vi "古田污水厂流程自动启动.vi"(11 "参数":cluster{"是否启用仪器":bool}) -> ()   [LabVIEW 2016, in "PLC.lvlib"]
uses:
  PLC.lvlib
panel:
  out "枚举":enum16{"初始化", "采配水启动", "等待", "配水", "排水", "结束"}(ring)
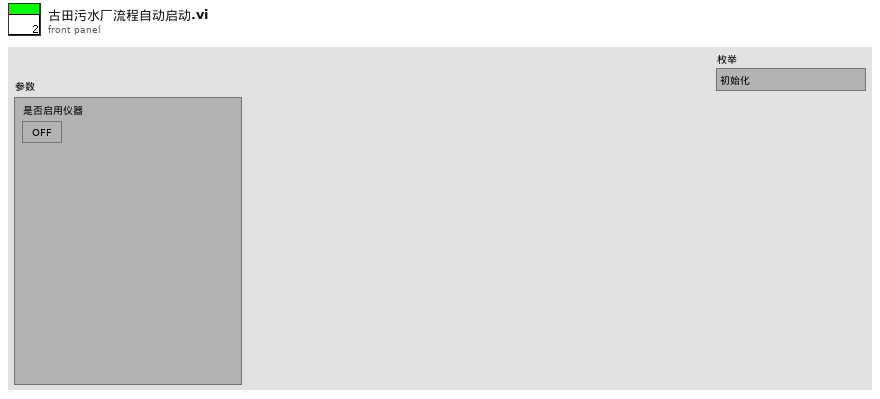
[diagram p1: front panel]
types:
  T1 = cluster{"命令":string, cluster{"starting address":u16, "holding register value":u16}}
  T2 = enum16{"待机", "启动氨氮", "氨氮测量中", "启动总磷", "总磷测量中", "结束"}
  T3 = cluster{"测量模式":enum16{"待机", "水样测试", "标样核查", "零点核查", "跨度核查", "空白测试", "平行样测试", "加标回收", "空白校准", "标样校准", "初始化（清洗）"}, "数据标记表":string, "测量时间":dbl}
  T4 = enum16{"待机", "水样测试", "标样核查", "零点核查", "跨度核查", "空白测试", "平行样测试", "加标回收", "空白校准", "标样校准", "初始化（清洗）"}
  T5 = cluster{"站号":u16, "量程切换":enum32{"H", "L", "AUTO"}, "控制命令":enum16{"启动测量", "标样核查", "零点核查", "跨度核查", "空白测试", "平行样测试", "加标回收", "空白校准", "标样校准", "初始化（清洗）", "停止测试", "仪器重启", "校时", "模式设置", "测量间隔设置", "盲样测试"}, "模式设置":enum16{"待机", "连续模式", "周期模式", "定点模式", "受控模式", "手动模式"}, "测量间隔":u16}
  T6 = cluster{"时间标识":timestamp, "设备":string, "日志信息":string}
  T7 = cluster{"R0":i16, "R1":i16, "R2":i16, "R3":i16, "R4":i16, "R5":i16, "R6":i16, "R7":i16, "R8":i16, "R9":i16, "R10":i16, "R11":i16, "R12":i16, "R13":i16, "R14":i16, "R15":i16, "R16":i16, "R17":i16, "R18":i16, "R19":i16}
  T8 = enum32{"Bad", "Idle", "Run top level", "Running"}
  T9 = cluster{"系统时间":timestamp, "工作状态":enum16{"空闲", "水样测试", "标样核查", "零点核查", "跨度核查", "空白测试", "平行样测试", "加标回收", "空白校准", "标样校准", "初始化（清洗）"}, "测量模式":enum16{"待机", "连续模式", "周期模式", "定点模式", "受控模式", "手动模式"}, "告警代码":enum16{"无告警", "缺试剂告警", "缺水样告警", "缺蒸馏水告警", "缺标液告警", "仪表漏液告警", "标定异常告警", "超量程告警", "加热异常", "低试剂预警", "超上限告警", "超下限告警", "仪表内部其他异常", "滴定异常告警", "电极异常告警", "量程切换告警", "参数设置告警", "PH电极电位异常", "电导率电极异常", "浊度光度异常", "溶解氧电极异常", "溶解氧光强异常", "温度异常告警", "PH异常告警", "溶解氧异常告警", "电导率异常告警", "浊度异常告警", "叶绿素异常告警", "藻密度异常告警", "蓝绿藻异常告警", "ORP异常告警", "氨氮异常告警", "清洁刷异常告警", "SD卡异常告警", "蓝牙异常告警", "Wifi异常告警", "流程异常告警"}, "故障代码":enum16{"无故障", "电机故障", "温度故障", "通讯故障", "滴定故障"}, "日志代码":u16, "软件版本":u16, "F0":sgl, "F1":sgl, "F2":sgl, "F3":sgl, "T":sgl, "H":sgl, "id":u16, "flowid":u16, "量程":u16}
  T10 = enum16{"空闲", "水样测试", "标样核查", "零点核查", "跨度核查", "空白测试", "平行样测试", "加标回收", "空白校准", "标样校准", "初始化（清洗）"}
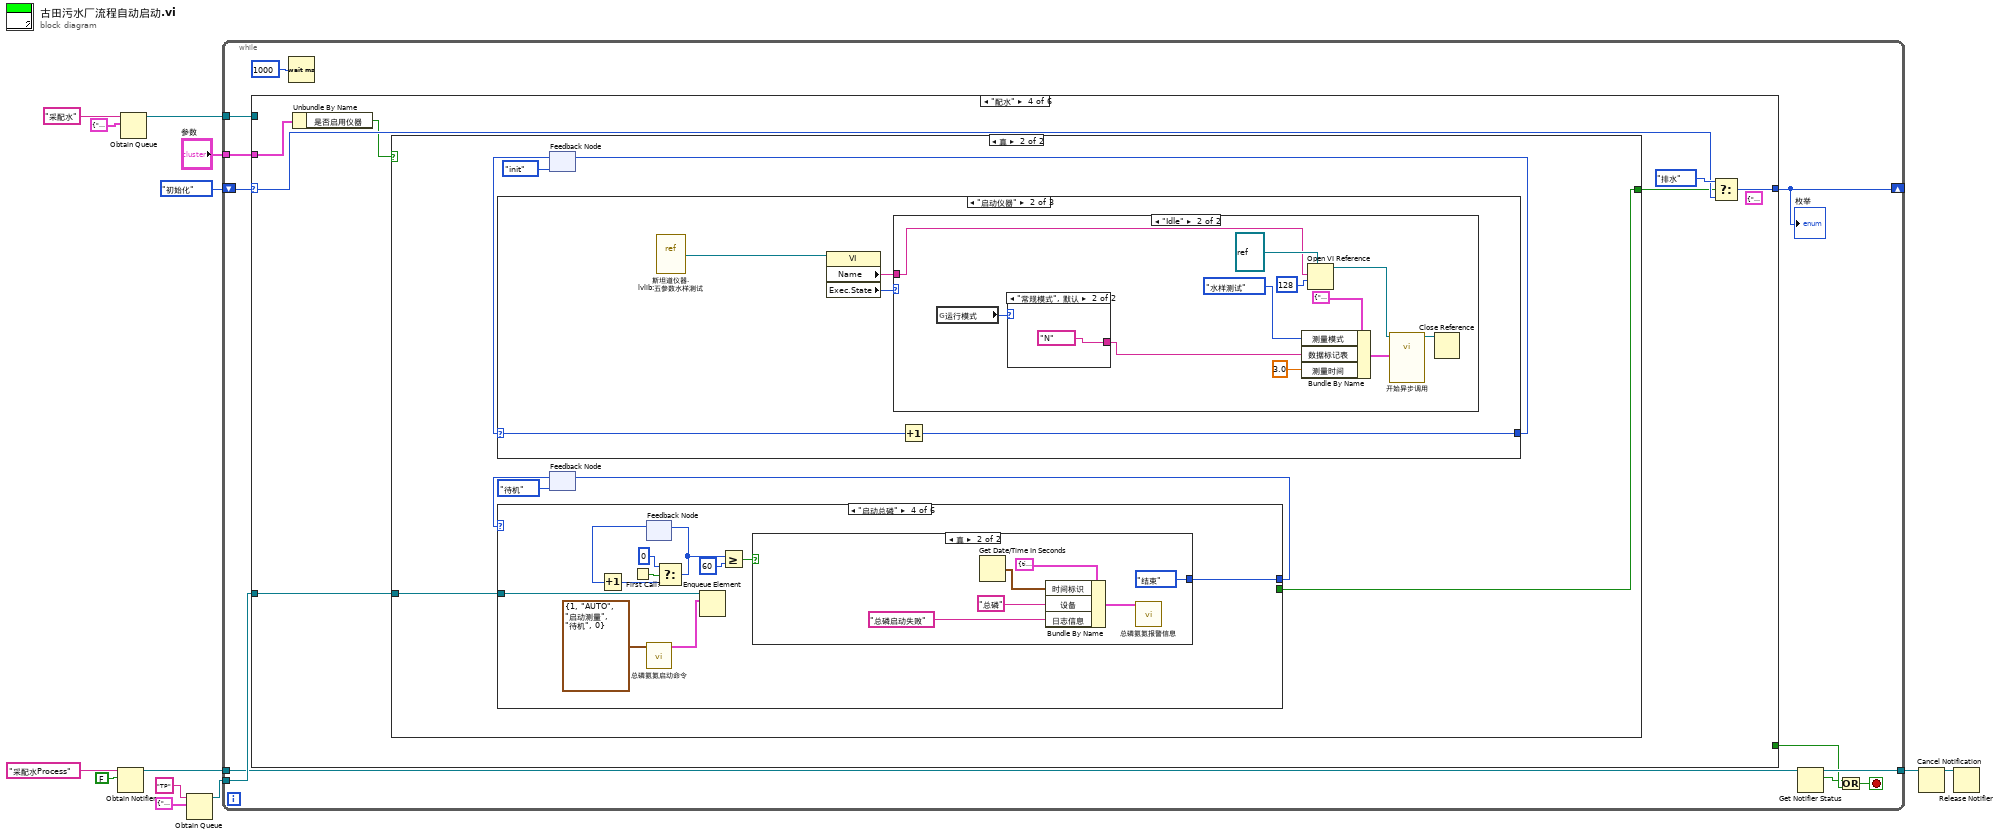
[diagram p0: block diagram]
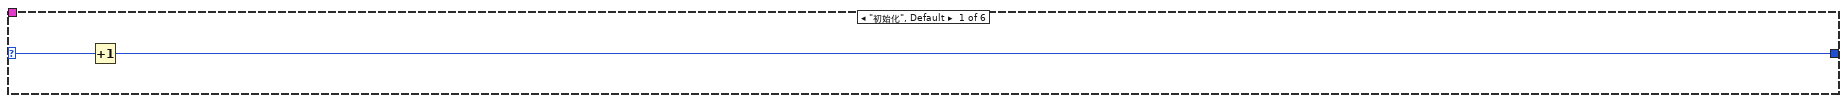
[diagram p2: hidden frame]
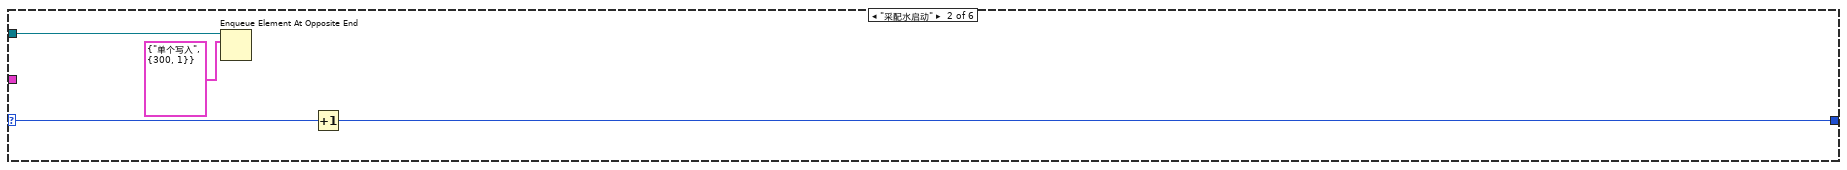
[diagram p3: hidden frame]
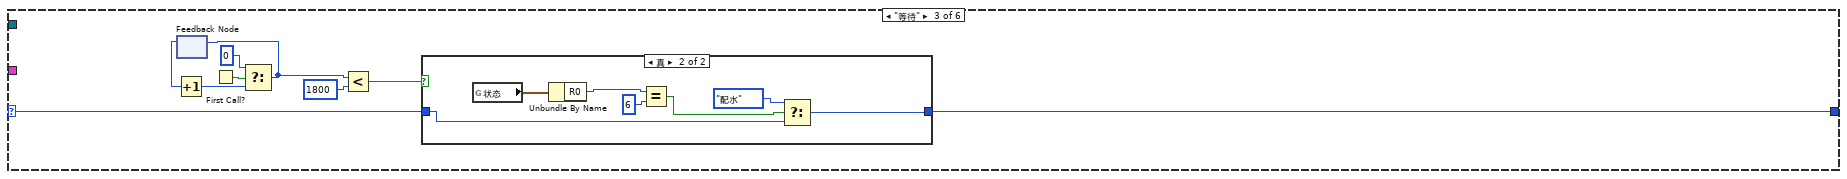
[diagram p4: hidden frame]
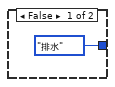
[diagram p5: hidden frame]
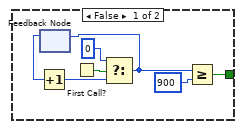
[diagram p6: hidden frame]
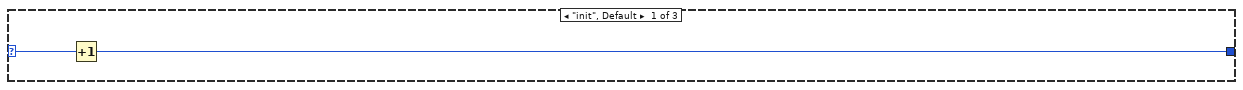
[diagram p7: hidden frame]
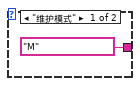
[diagram p9: hidden frame]
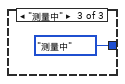
[diagram p10: hidden frame]
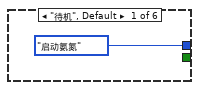
[diagram p11: hidden frame]
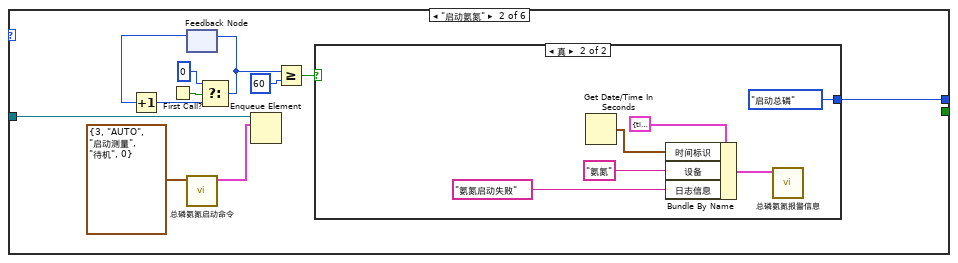
[diagram p12: hidden frame]
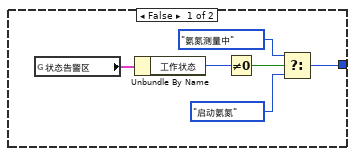
[diagram p13: hidden frame]
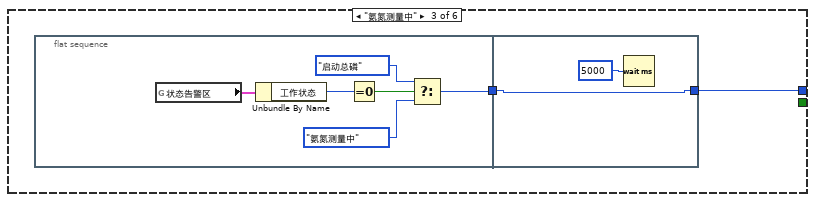
[diagram p14: hidden frame]
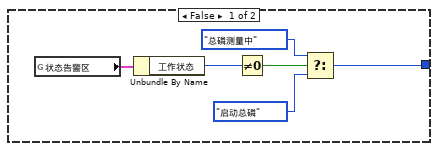
[diagram p15: hidden frame]
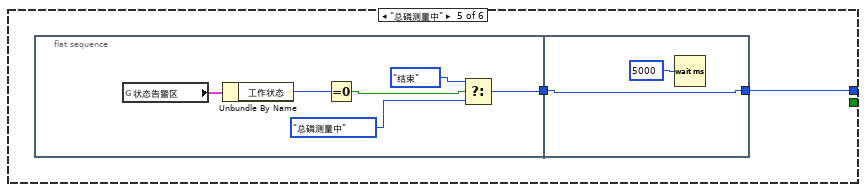
[diagram p16: hidden frame]
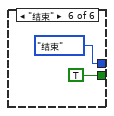
[diagram p17: hidden frame]
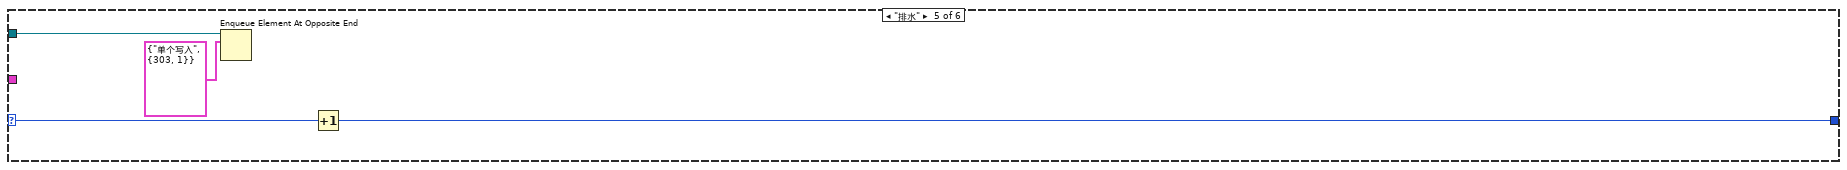
[diagram p18: hidden frame]
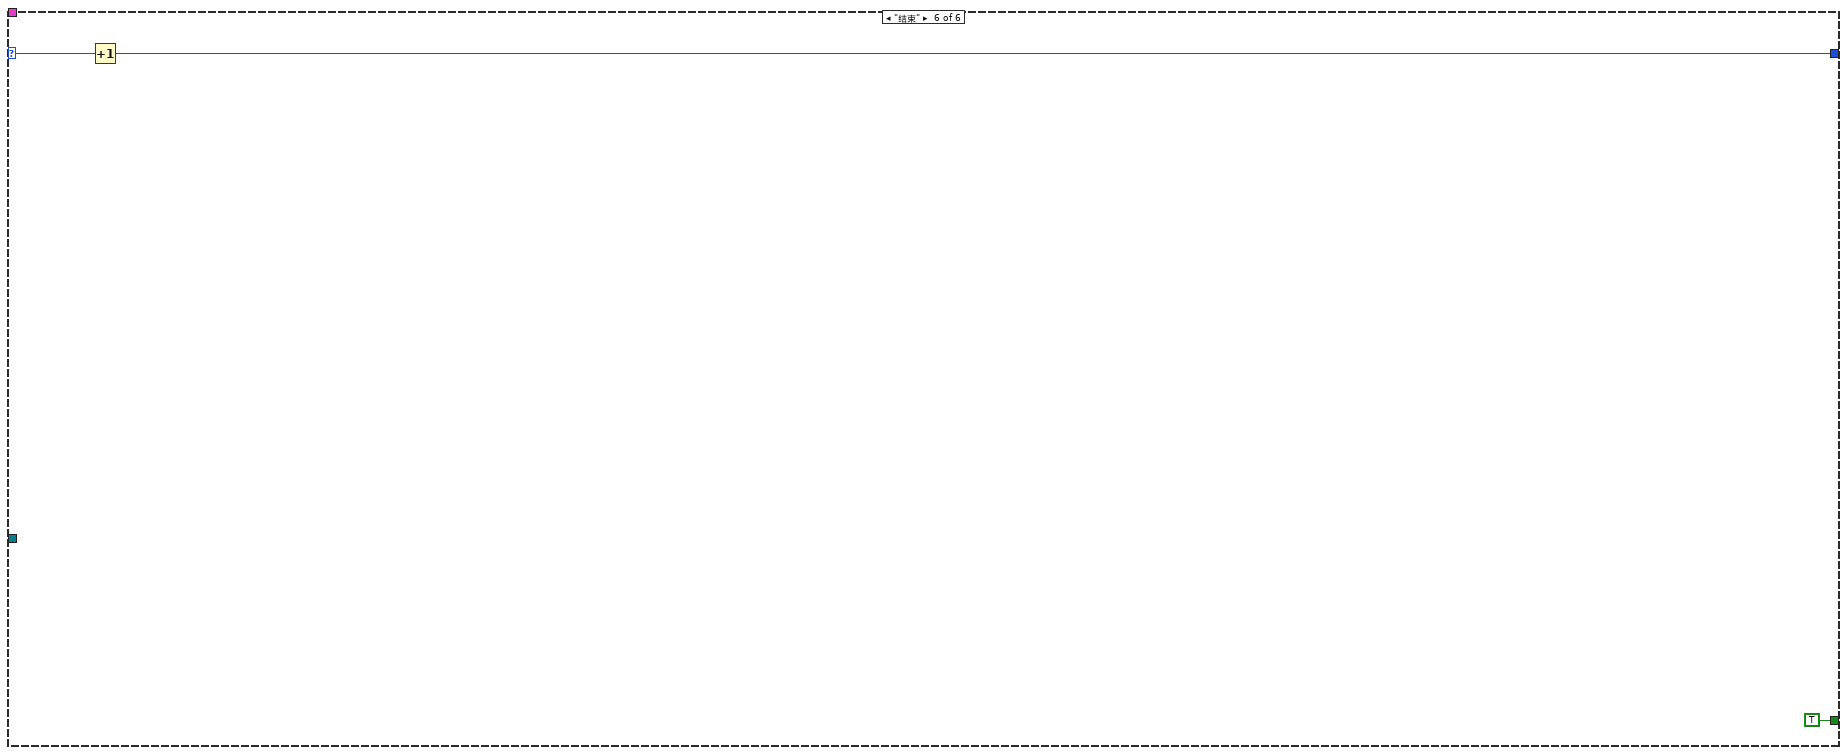
[diagram p19: hidden frame]
diagram:
  n1 = Obtain Notifier(name (unnamed)="采配水Process" ("名称（未命名）"), notification data type=FALSE) -> (notifier out=w3:refnum<notifier>)  [unwired: 2 in, 2 out]
  n2 = Obtain Queue(name (unnamed)="采配水" ("名称（未命名）"), element data type=cluster{"命令":string, "数据":variant} {"命令"="", "数据"=variant}) -> (queue out=w11:refnum<queue>)  [unwired: 3 in, 2 out]
  n3 = Obtain Queue(name (unnamed)="TP" ("名称（未命名）"), element data type=cluster{"命令":string, "data":variant} {"命令"="", "data"=variant}) -> (queue out=w7:refnum<queue>)  [unwired: 3 in, 2 out]
  n4 = while {
    tunnel: w11 -> [w24]
    shift-right: [w22] -> _
    shift-left: enum16{"初始化", "采配水启动", "等待", "配水", "排水", "结束"}."初始化" ("枚举") -> [w23]
    tunnel: w7 -> [w20]
    tunnel: "参数" -> [w19]
    tunnel: w3 -> [w18]
    tunnel: [w17] -> w2
    stop <- w16 stop-if-true
    n5 = case shown="\"配水\"" w23 {
      selector: w23 -> [w26 w28 w37 w53 w161 w166]
      tunnel: w24 -> [_ w29 _ _ w162 _]
      tunnel: [w25 w27 w36 w52 w160 w165] -> w22
      tunnel: [_ _ _ _ _ TRUE] -> w15
      tunnel: w20 -> [_ _ _ w51 _ _]
      tunnel: w19 -> [_ _ _ w50 _ _]
      frame "初始化", Default {
        n6 = Increment(x=w26) -> (x+1=w25:enum16{"初始化", "采配水启动", "等待", "配水", "排水", "结束"})
      }
      frame "采配水启动" {
        n7 = Enqueue Element At Opposite End(queue=w29, element=T1 {"命令"="单个写入", {"starting address"=300, "holding register value"=1}} ("元素")) -> ()  [unwired: 2 in, 3 out]
        n8 = Increment(x=w28) -> (x+1=w27:enum16{"初始化", "采配水启动", "等待", "配水", "排水", "结束"})
      }
      frame "等待" {
        n9 = feedback #1() -> (w33:i32)  [unwired: 1 in]
        n10 = Increment(x=w33) -> (x+1=w32:i32)
        n11 = First Call?() -> (First Call?: T/F=w34:bool)
        n12 = Select(t=0, s=w34, f=w32) -> (s? t:f=w31:i32)
        n13 = feedback-in #1(w31) -> ()
        n14 = Less?(x=w31, y=1800) -> (x < y?=w38:bool)
        n15 = case shown="真" w38 {
          tunnel: w37 -> [_ w42]
          tunnel: [enum16{"初始化", "采配水启动", "等待", "配水", "排水", "结束"}."排水" ("枚举") w41] -> w36
          frame False {
          }
          frame True {
            n16 = global read "采配水全局变量.vi" "状态"() -> (w47:T7)
            n17 = Unbundle By Name(w47) -> ("R0"=w46:i16)
            n18 = Equal?(x=w46, y=i16 6) -> (x = y?=w44:bool)
            n19 = Select(t=enum16{"初始化", "采配水启动", "等待", "配水", "排水", "结束"}."配水" ("枚举"), s=w44, f=w42) -> (s? t:f=w41:enum16{"初始化", "采配水启动", "等待", "配水", "排水", "结束"})
          }
        }
      }
      frame "配水" {
        (unwired) cluster{"命令":string, "data":variant} {"命令"="启动", "data"=variant(cluster{"站号":u16, "控制命令输出":u16[]} {"站号"=1, "控制命令输出"=[256, 0]})} ("元素")
        n20 = Unbundle By Name(w50) -> ("是否启用仪器"=w49:bool)
        n21 = case shown="真" w49 {
          tunnel: w51 -> [_ w66]
          tunnel: [w55 w65] -> w48
          frame False {
            n22 = feedback #2() -> (w59:i32)  [unwired: 1 in]
            n23 = Increment(x=w59) -> (x+1=w58:i32)
            n24 = First Call?() -> (First Call?: T/F=w60:bool)
            n25 = Select(t=0, s=w60, f=w58) -> (s? t:f=w56:i32)
            n26 = feedback-in #2(w56) -> ()
            n27 = Greater Or Equal?(x=w56, y=900) -> (x >= y?=w55:bool)
          }
          frame True {
            n28 = feedback #3(enum16{"init", "启动仪器", "测量中"}."init") -> (w63:enum16{"init", "启动仪器", "测量中"})
            n29 = case shown="\"启动仪器\"" w63 {
              selector: w63 -> [w71 w76 _]
              tunnel: [w70 w75 enum16{"init", "启动仪器", "测量中"}."测量中"] -> w64
              frame "init", Default {
                n30 = Increment(x=w71) -> (x+1=w70:enum16{"init", "启动仪器", "测量中"})
              }
              frame "启动仪器" {
                n31 = vi-ref "斯坦道仪器.lvlib:五参数水样测试.vi"() -> (w73:refnum<vi>)
                n32 = property class="VI"(reference=w73) -> ("Name"=w72:string, "Exec.State"=w74:T8)  [unwired: 1 in, 2 out]
                n33 = case shown="\"Idle\"" w74 {
                  tunnel: w72 -> [_ w83]
                  frame "Bad", Default {
                  }
                  frame "Idle" {
                    n34 = global read "系统变量.vi" "运行模式"() -> (w78:enum16{"维护模式", "常规模式", "应急模式", "质控模式"})
                    n35 = case shown="\"常规模式\", 默认" w78 {
                      tunnel: ["M" ("数据标记表") "N" ("数据标记表")] -> w77
                      frame "维护模式" {
                      }
                      frame "常规模式", Default {
                      }
                    }
                    n36 = Bundle By Name(cluster=T3 {"测量模式"=enum."待机", "数据标记表"="", "测量时间"=0.0} ("启动参数"), "测量模式"=T4."水样测试", "数据标记表"=w77, "测量时间"=3.0) -> (w79:T3)
                    n37 = Open VI Reference(type specifier VI Refnum (for type only)=refnum<vi> refnum ("类型说明符VI引用句柄（仅用于类型）"), vi path=w83, options=128 ("选项")) -> (vi reference=w82:refnum<vi>)  [unwired: 3 in, 1 out]
                    n38 = call-by-ref "开始异步调用"(reference=w82, "启动参数"=w79) -> (reference out=w81:refnum<vi>)  [unwired: 12 in, 1 out]
                    n39 = Close Reference(reference=w81) -> ()  [unwired: 1 in, 1 out]
                  }
                }
                n40 = Increment(x=w76) -> (x+1=w75:enum16{"init", "启动仪器", "测量中"})
              }
              frame "测量中" {
              }
            }
            n41 = feedback-in #3(w64) -> ()
            n42 = feedback #4(T2."待机") -> (w68:T2)
            n43 = case shown="\"启动总磷\"" w68 {
              tunnel: [T2."启动氨氮" w101 w116 w134 w149 T2."结束"] -> w67
              tunnel: w66 -> [_ w102 _ w135 _ _]
              tunnel: [_ _ _ _ _ TRUE] -> w65
              frame "待机", Default {
              }
              frame "启动氨氮" {
                n44 = First Call?() -> (First Call?: T/F=w99:bool)
                n45 = feedback #5() -> (w98:i32)  [unwired: 1 in]
                n46 = Increment(x=w98) -> (x+1=w97:i32)
                n47 = call "总磷氨氮启动命令.vi"("参数"=T5 {"站号"=3, "量程切换"=enum."AUTO", "控制命令"=enum."启动测量", "模式设置"=enum."待机", "测量间隔"=0}) -> ("启动命令"=w93:cluster{"命令":string, "data":variant})  [unwired: 10 in]
                n48 = Select(t=0, s=w99, f=w97) -> (s? t:f=w96:i32)
                n49 = feedback-in #5(w96) -> ()
                n50 = Enqueue Element(queue=w102, element=w93) -> ()  [unwired: 2 in, 3 out]
                n51 = Greater Or Equal?(x=w96, y=60) -> (x >= y?=w94:bool)
                n52 = case shown="真" w94 {
                  tunnel: [w105 T2."启动总磷"] -> w101
                  frame False {
                    n53 = global read "VAR总磷氨氮全局变量.vi" "状态告警区"() -> (w108:T9)
                    n54 = Unbundle By Name(w108) -> ("工作状态"=w107:T10)
                    n55 = Not Equal To 0?(x=w107) -> (x != 0?=w106:bool)
                    n56 = Select(t=T2."氨氮测量中", s=w106, f=T2."启动氨氮") -> (s? t:f=w105:T2)
                  }
                  frame True {
                    n57 = Get Date/Time In Seconds() -> (seconds since 1Jan1904=w113:timestamp)
                    n58 = Bundle By Name(cluster=T6 {"时间标识"=timestamp(0 s since 1904-01-01), "设备"="", "日志信息"=""} ("data in"), "时间标识"=w113, "设备"="氨氮", "日志信息"="氨氮启动失败") -> (w109:T6)
                    n59 = call "总磷氨氮报警信息.vi"("data in"=w109) -> ()  [unwired: 11 in]
                  }
                }
              }
              frame "氨氮测量中" {
                n60 = flat-sequence {
                  tunnel: [w120] -> w115
                  tunnel: [w124] -> w116
                  tunnel: w115 -> [w124]
                  frame #0 {
                    n61 = global read "VAR总磷氨氮全局变量.vi" "状态告警区"() -> (w121:T9)
                    n62 = Unbundle By Name(w121) -> ("工作状态"=w122:T10)
                    n63 = Equal To 0?(x=w122) -> (x = 0?=w119:bool)
                    n64 = Select(t=T2."启动总磷", s=w119, f=T2."氨氮测量中") -> (s? t:f=w120:T2)
                  }
                  frame #1 {
                    n65 = Wait (ms)(milliseconds to wait=u32 5000 ("等待时间（毫秒）")) -> ()  [unwired: 1 out]
                  }
                }
              }
              frame "启动总磷" {
                n66 = First Call?() -> (First Call?: T/F=w132:bool)
                n67 = feedback #6() -> (w131:i32)  [unwired: 1 in]
                n68 = Increment(x=w131) -> (x+1=w130:i32)
                n69 = call "总磷氨氮启动命令.vi"("参数"=T5 {"站号"=1, "量程切换"=enum."AUTO", "控制命令"=enum."启动测量", "模式设置"=enum."待机", "测量间隔"=0}) -> ("启动命令"=w126:cluster{"命令":string, "data":variant})  [unwired: 10 in]
                n70 = Select(t=0, s=w132, f=w130) -> (s? t:f=w129:i32)
                n71 = feedback-in #6(w129) -> ()
                n72 = Enqueue Element(queue=w135, element=w126) -> ()  [unwired: 2 in, 3 out]
                n73 = Greater Or Equal?(x=w129, y=60) -> (x >= y?=w127:bool)
                n74 = case shown="真" w127 {
                  tunnel: [w138 T2."结束"] -> w134
                  frame False {
                    n75 = global read "VAR总磷氨氮全局变量.vi" "状态告警区"() -> (w139:T9)
                    n76 = Unbundle By Name(w139) -> ("工作状态"=w140:T10)
                    n77 = Not Equal To 0?(x=w140) -> (x != 0?=w141:bool)
                    n78 = Select(t=T2."总磷测量中", s=w141, f=T2."启动总磷") -> (s? t:f=w138:T2)
                  }
                  frame True {
                    n79 = Get Date/Time In Seconds() -> (seconds since 1Jan1904=w147:timestamp)
                    n80 = Bundle By Name(cluster=T6 {"时间标识"=timestamp(0 s since 1904-01-01), "设备"="", "日志信息"=""} ("data in"), "时间标识"=w147, "设备"="总磷", "日志信息"="总磷启动失败") -> (w143:T6)
                    n81 = call "总磷氨氮报警信息.vi"("data in"=w143) -> ()  [unwired: 11 in]
                  }
                }
              }
              frame "总磷测量中" {
                n82 = flat-sequence {
                  tunnel: [w153] -> w148
                  tunnel: [w157] -> w149
                  tunnel: w148 -> [w157]
                  frame #0 {
                    n83 = global read "VAR总磷氨氮全局变量.vi" "状态告警区"() -> (w154:T9)
                    n84 = Unbundle By Name(w154) -> ("工作状态"=w155:T10)
                    n85 = Equal To 0?(x=w155) -> (x = 0?=w152:bool)
                    n86 = Select(t=T2."结束", s=w152, f=T2."总磷测量中") -> (s? t:f=w153:T2)
                  }
                  frame #1 {
                    n87 = Wait (ms)(milliseconds to wait=u32 5000 ("等待时间（毫秒）")) -> ()  [unwired: 1 out]
                  }
                }
              }
              frame "结束" {
              }
            }
            n88 = feedback-in #4(w67) -> ()
          }
        }
        n89 = Select(t=enum16{"初始化", "采配水启动", "等待", "配水", "排水", "结束"}."排水" ("枚举"), s=w48, f=w53) -> (s? t:f=w52:enum16{"初始化", "采配水启动", "等待", "配水", "排水", "结束"})
      }
      frame "排水" {
        n90 = Enqueue Element At Opposite End(queue=w162, element=T1 {"命令"="单个写入", {"starting address"=303, "holding register value"=1}} ("元素")) -> ()  [unwired: 2 in, 3 out]
        n91 = Increment(x=w161) -> (x+1=w160:enum16{"初始化", "采配水启动", "等待", "配水", "排水", "结束"})
      }
      frame "结束" {
        n92 = Increment(x=w166) -> (x+1=w165:enum16{"初始化", "采配水启动", "等待", "配水", "排水", "结束"})
      }
    }
    "枚举" <- w22
    n93 = Wait (ms)(milliseconds to wait=u32 1000 ("等待时间（毫秒）")) -> ()  [unwired: 1 out]
    n94 = Get Notifier Status(notifier=w18) -> (notifier out=w17:refnum<notifier>, current notification=w14:bool)  [unwired: 1 in, 3 out]
    n95 = Or(x=w14, y=w15) -> (x .or. y?=w16:bool)
  }
  n96 = Cancel Notification(0:w2) -> (8:w1:refnum<notifier>)  [unwired: 1 in, 2 out]
  n97 = Release Notifier(notifier=w1) -> ()  [unwired: 2 in, 3 out]
